vi "FreqPwrMeasureExample.vi"() -> ()   [LabVIEW 2015]
uses:
  PhyPort.ctl
  PwrFreq.ctl
  VISAOperation.ctl
panel:
  in  "PathlossConfig":T2={"PathlossFilePath"=path "D:/WTM and WTS training/WLAN Solutions/Pathloss/External Pathloss.txt", "Pathloss Table Name"="wlan", "PhyPort"=enum."Port6"}
  in  "Freq/Pwr":T3
  in  "MeasureConfig":T4={"TriggerSource"=enum."RIO0", "ReferenceLevel"=0.0, "Freq"=5180000000.0, "PhyPort"=enum."Port6"}
  out "Results":string="0.08\n"
  in  "VISA resource name":refnum<visa-resource-name>="TCPIP0::10.144.41.39::inst0::INSTR"
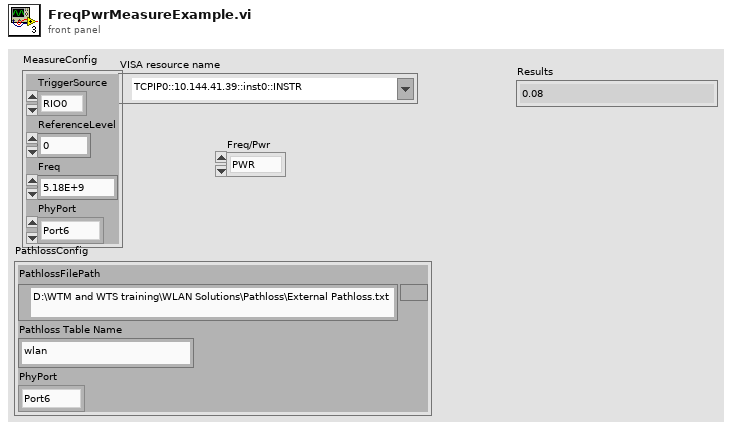
[diagram p1: front panel]
types:
  T1 = typedef "PhyPort.ctl" = enum16{"Port0", "Port1", "Port2", "Port3", "Port4", "Port5", "Port6", "Port7"}
  T2 = cluster{"PathlossFilePath":path, "Pathloss Table Name":string, "PhyPort":T1}
  T3 = typedef "PwrFreq.ctl" = enum16{"PWR", "FREQ"}
  T4 = cluster{"TriggerSource":enum16{"RIO0", "RIO1"}, "ReferenceLevel":dbl, "Freq":dbl, "PhyPort":T1}
  T5 = typedef "VISAOperation.ctl" = enum16{"RunFile", "OpenDebugPanel", "ReadError", "ReadSTB", "Reset", "Clean", "CloseVISA", "RunCMD", "OpenVISA"}
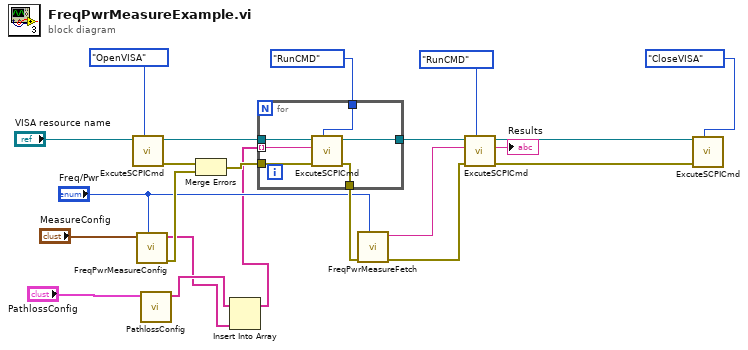
[diagram p0: block diagram]
diagram:
  n1 = call "ExcuteSCPICmd.vi"("VISAOperation"=VISAOperation."OpenVISA", "VISA resource name"="VISA resource name") -> ("error out"=w18:errorcluster, "reference out"=w17:refnum<visa-resource-name>)  [unwired: 6 in, 2 out]
  n2 = call "FreqPwrMeasureConfig.vi"("Freq/Pwr"="Freq/Pwr", "FreqMeasureConfig"="MeasureConfig") -> ("error out"=w9:errorcluster, "FreqMeasureConfig"=w2:string[])  [unwired: 8 in]
  n3 = call "PathlossConfig.vi"("PathlossConfig"="PathlossConfig") -> ("PahtlossCMD"=w3:string[])  [unwired: 9 in, 1 out]
  n4 = Merge Errors(w18, w9) -> (w14:errorcluster)
  n5 = Insert Into Array(array=w3, new element=w2) -> (w1:string[])  [unwired: 1 in]
  n6 = for {
    tunnel: VISAOperation."RunCMD" ("VISAOperation") -> [w26]
    tunnel: w17 -> [w28]
    tunnel: [w27] -> w16
    tunnel: w1 -> [w25] mode=indexing
    tunnel: w14 -> [w24]
    tunnel: [w23] -> w8
    n7 = call "ExcuteSCPICmd.vi"("VISAOperation"=w26, "error in (no error)"=w24, "Run Command"=w25, "VISA resource name"=w28) -> ("error out"=w23:errorcluster, "reference out"=w27:refnum<visa-resource-name>)  [unwired: 4 in, 2 out]
  }
  n8 = call "FreqPwrMeasureFetch.vi"("Freq/Pwr"="Freq/Pwr", "error in (no error)"=w8) -> ("error out"=w7:errorcluster, "FreqFetchCMD"=w11:string)  [unwired: 8 in]
  n9 = call "ExcuteSCPICmd.vi"("VISAOperation"=VISAOperation."RunCMD", "error in (no error)"=w7, "Run Command"=w11, "VISA resource name"=w16) -> ("error out"=w12:errorcluster, "Results"=→"Results":string, "reference out"=w13:refnum<visa-resource-name>)  [unwired: 4 in, 1 out]
  n10 = call "ExcuteSCPICmd.vi"("VISAOperation"=VISAOperation."CloseVISA", "error in (no error)"=w12, "VISA resource name"=w13) -> ()  [unwired: 5 in, 4 out]
